vi "Subscribe and unsubscribe to CAM.vi"(8 "error in (no error)":errorcluster, 9 "Sub T/ Unsub F":bool, 10 "Subscriber Data":T1, 11 "Camera Queue":refnum<queue>) -> (0 "error out":errorcluster, 3 "Camera queue out":refnum<queue>)   [LabVIEW 2024, in "RSeries_CAM.lvlib"]
uses:
  RSeries_CAM.lvlib
  ARCH/Message Queue/Message Cluster.ctl
  ARCH/Message Queue/Message Queue.lvlib
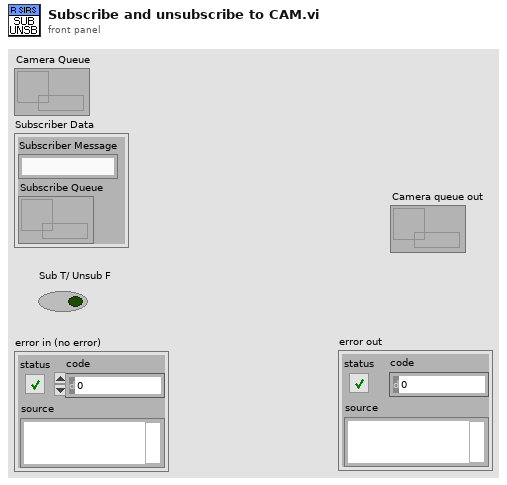
[diagram p1: front panel]
types:
  T1 = cluster{"Subscriber Message":string, "Subscribe Queue":refnum<queue>}
  T2 = typedef "Message Queue.lvlib/Message Cluster.ctl" = cluster{"Message":string, "Message Data":variant}
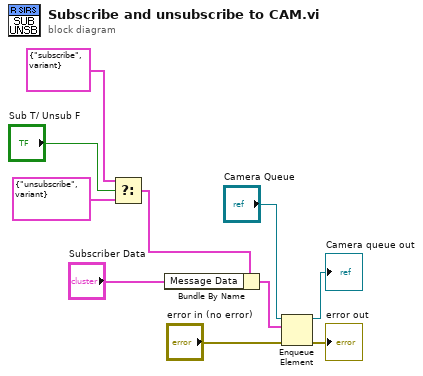
[diagram p0: block diagram]
diagram:
  n1 = Select(t=T2 {"Message"="subscribe", "Message Data"=variant} ("element"), s="Sub T/ Unsub F", f=T2 {"Message"="unsubscribe", "Message Data"=variant} ("element")) -> (s? t:f=w5:T2)
  n2 = Bundle By Name(cluster=w5, "Message Data"="Subscriber Data") -> (w4:T2)
  n3 = Enqueue Element(queue="Camera Queue", element=w4, error in (no error)="error in (no error)") -> (queue out=→"Camera queue out":refnum<queue>, error out=→"error out":errorcluster)  [unwired: 1 in, 1 out]
